vi "sv_Prepare STFT blocks [indices].vi"(0 "scaled signal [EU]":waveform(dbl), 3 "FFT block size":i32=1024 min=1, 5 "error in (no error)":errorcluster, 9 "indices":i32) -> (14 "scaled signal [EU]":waveform(dbl), 19 "error out":errorcluster)   [LabVIEW 2017]
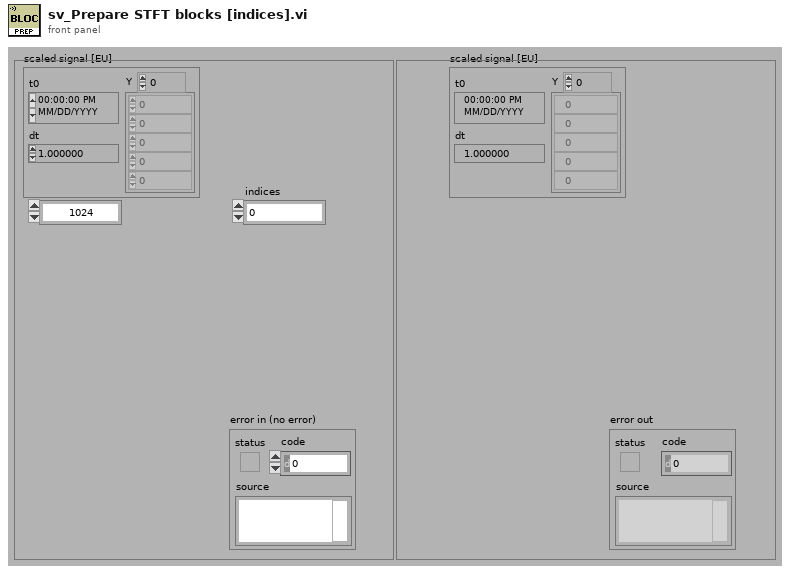
[diagram p1: front panel]
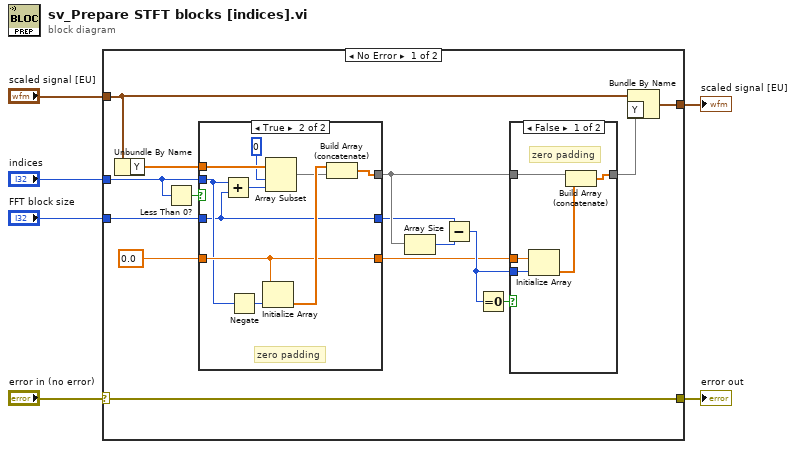
[diagram p0: block diagram]
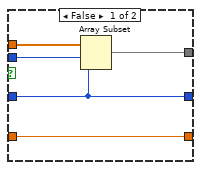
[diagram p2: hidden frame]
diagram:
  n1 = case shown="No Error" "error in (no error)" {
    selector: "error in (no error)" -> [w12 w43]
    tunnel: "FFT block size" -> [w8 _]
    tunnel: "indices" -> [w15 _]
    tunnel: "scaled signal [EU]" -> [w14 w44]
    tunnel: [w12 w43] -> w2
    tunnel: [w11 w44] -> w1
    frame No Error {
      n2 = Unbundle By Name(w14) -> ("Y"=w13:dbl[])
      n3 = Less Than 0?(x=w15) -> (x < 0?=w18:bool)
      n4 = case shown="True" w18 {
        tunnel: w15 -> [w25 w28]
        tunnel: w13 -> [w26 w35]
        tunnel: w8 -> [w23 w27]
        tunnel: [w24 w30] -> w16
        tunnel: 0.0 -> [w22 w29]
        tunnel: [w23 w27] -> w9
        tunnel: [w22 w29] -> w7
        frame False {
          n5 = Array Subset(array=w26, index=w25, length=w23) -> (w24:dbl[])
        }
        frame True {
          # "zero padding"
          n6 = Add(x=w28, y=w27) -> (x+y=w33:i32)
          n7 = Negate(x=w28) -> (-x=w36:i32)
          n8 = Initialize Array(w29, w36) -> (w32:dbl[])
          n9 = Array Subset(array=w35, index=0, length=w33) -> (w31:dbl[])
          n10 = Build Array (concatenate)(w32, w31) -> (w30:dbl[])
        }
      }
      n11 = Array Size(array=w16) -> (size(s)=w19:i32)
      n12 = Subtract(x=w9, y=w19) -> (x-y=w17:i32)
      n13 = Equal To 0?(x=w17) -> (x = 0?=w20:bool)
      n14 = case shown="False" w20 {
        tunnel: [w38 w42] -> w21
        tunnel: w16 -> [w41 w42]
        tunnel: w17 -> [w40 _]
        tunnel: w7 -> [w37 _]
        frame False {
          # "zero padding"
          n15 = Initialize Array(w37, w40) -> (w39:dbl[])
          n16 = Build Array (concatenate)(w41, w39) -> (w38:dbl[])
        }
        frame True {
        }
      }
      n17 = Bundle By Name(cluster=w14, "Y"=w21) -> (w11:waveform(dbl))
    }
    frame Error {
    }
  }
  "error out" <- w2
  "scaled signal [EU]" <- w1
